vi "grab.vi"(8 "error in (no error)":errorcluster, 11 "camera in":refnum<class "camera.lvclass">) -> (0 "error out":errorcluster, 2 "Image Out":T1, 3 "camera out":refnum<class "camera.lvclass">)   [LabVIEW 2017, in "camera.lvclass"]
uses:
  camera.lvclass
  <vilib>/vision/Image Controls.llb/IMAQ Image.ctl
  <vilib>/vision/driver/IMAQdx.llb/IMAQdx Buffer Number Mode.ctl
  <vilib>/vision/driver/NI_Vision_Acquisition_Software.lvlib
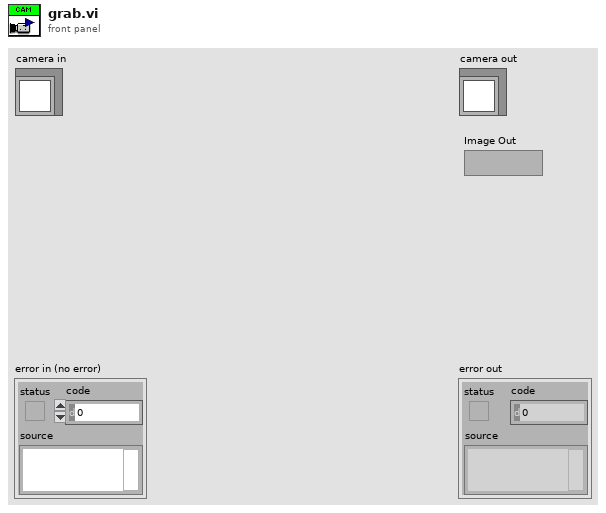
[diagram p1: front panel]
types:
  T1 = typedef "IMAQ Image.ctl" = refnum<image>
  T2 = typedef "NI_Vision_Acquisition_Software.lvlib/IMAQdx Buffer Number Mode.ctl" = enum32{"Next", "Last", "Buffer Number", "Every", "Last New"}
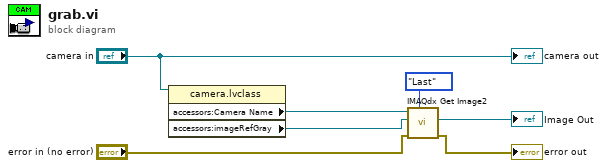
[diagram p0: block diagram]
diagram:
  n1 = property class="camera.lvclass"(reference="camera in") -> ("accessors:Camera Name"=w6:refnum<k21>, "accessors:imageRefGray"=w2:T1)  [unwired: 1 in, 2 out]
  n2 = call <vilib>:"IMAQdx Get Image2.vi"("Buffer Number Mode (Next)"=IMAQdx_Buffer_Number_Mode."Last", "error in"="error in (no error)", "Image In"=w2, "Session In"=w6) -> ("error out"=→"error out":errorcluster, "Image Out"=→"Image Out":T1)  [unwired: 4 in, 2 out]
  "camera out" <- "camera in"
